vi "Destroy_LV_INI_Token.vi"   [LabVIEW 2020]
uses:
  <vilib>/Wiresmith Technology/G CLI/CLI Class/CLI.lvclass
  <vilib>/Utility/config.llb/NI_LVConfig.lvlib
types:
  T1 = enum32{"Invalid", "Standard", "Closed", "Hidden", "Minimized", "Maximized"}
  T2 = typedef "NI_LVConfig.lvlib/Config Data RefNum.ctl" = refnum<k1>
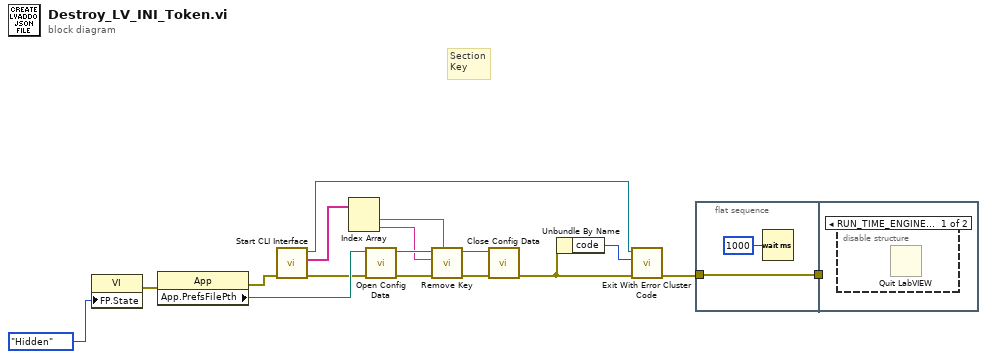
[diagram p0: block diagram]
diagram:
  # "Section\nKey"
  n1 = property class="VI"("FP.State"=T1."Hidden" ("Front Panel Window:State")) -> (error out=w14:errorcluster)  [unwired: 2 in, 1 out]
  n2 = property class="App"(error in=w14) -> (error out=w10:errorcluster, "App.PrefsFilePth"=w15:path)  [unwired: 1 in, 1 out]
  n3 = call <vilib>:"Start CLI Interface.vi"("error in (no error)"=w10) -> ("error out"=w11:errorcluster, "Custom Parameters"=w9:string[], "CLI out"=w16:refnum<class "CLI.lvclass">)  [unwired: 7 in, 1 out]
  n4 = Index Array(array=w9) -> (element #1=w4:string, element #2=w3:string)  [unwired: 2 in]
  n5 = call <vilib>:"Open Config Data.vi"("error in (no error)"=w11, "configuration file path"=w15) -> ("error out"=w8:errorcluster, "refnum"=w6:T2)  [unwired: 7 in, 1 out]
  n6 = call <vilib>:"Remove Key.vi"("section"=w4, "error in (no error)"=w8, "key"=w3, "refnum"=w6) -> ("error out"=w7:errorcluster, "refnum out"=w5:T2)  [unwired: 5 in, 1 out]
  n7 = call <vilib>:"Close Config Data.vi"("error in (no error)"=w7, "refnum"=w5) -> ("error out"=w13:errorcluster)  [unwired: 8 in, 1 out]
  n8 = Unbundle By Name(w13) -> ("code"=w12:i32)
  n9 = call <vilib>:"Exit With Error Cluster Code.vi"("error in (no error)"=w13, "No Error Code (0)"=w12, "CLI in"=w16) -> ("error out"=w1:errorcluster)  [unwired: 8 in]
  n10 = flat-sequence {
    tunnel: w1 -> [w19]
    tunnel: [w19] -> w2
    tunnel: w2 -> [_]
    frame #0 {
      n11 = Wait (ms)(milliseconds to wait=u32 1000) -> ()  [unwired: 1 out]
    }
    frame #1 {
      n12 = disable-structure shown="RUN_TIME_ENGINE==True" {
        frame condition #0 {
          n13 = Quit LabVIEW() -> ()  [unwired: 1 in]
        }
        frame condition #1 (active) {
        }
      }
    }
  }
